vi "Auto Climb Loop.vi"() -> (1 "Winch Out":dbl, 2 "Fire":bool, 3 "Extend":bool)   [LabVIEW 2015]
uses:
  Common Code/Climb Presets.ctl
panel:
  in  "Climb Presets":T1
  in  "Climb?":bool=TRUE
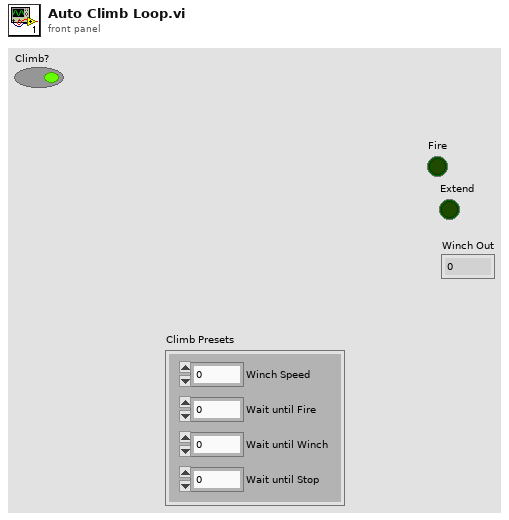
[diagram p1: front panel]
types:
  T1 = typedef "Climb Presets.ctl" = cluster{"Winch Speed":dbl, "Wait until Fire":dbl, "Wait until Winch":dbl, "Wait until Stop":dbl}
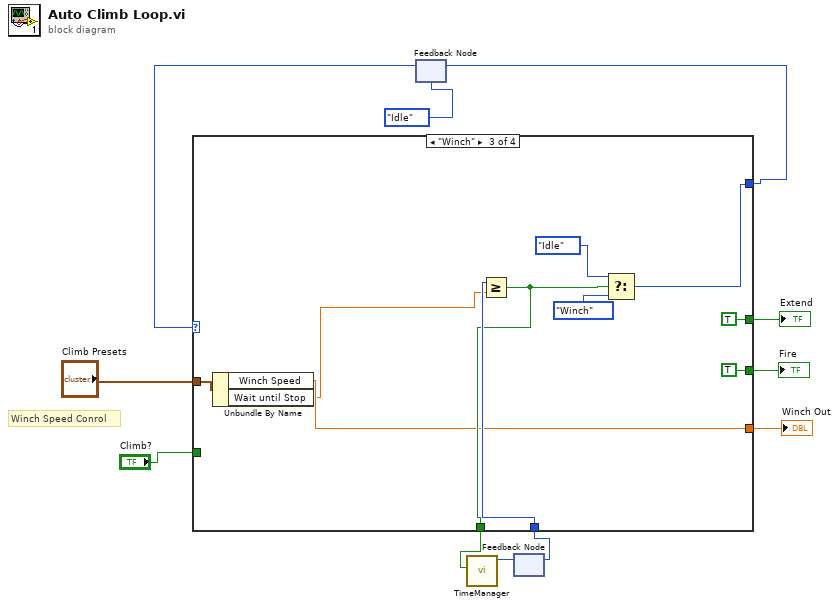
[diagram p0: block diagram]
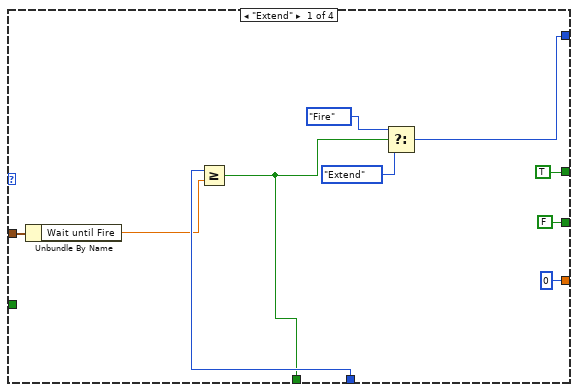
[diagram p2: hidden frame]
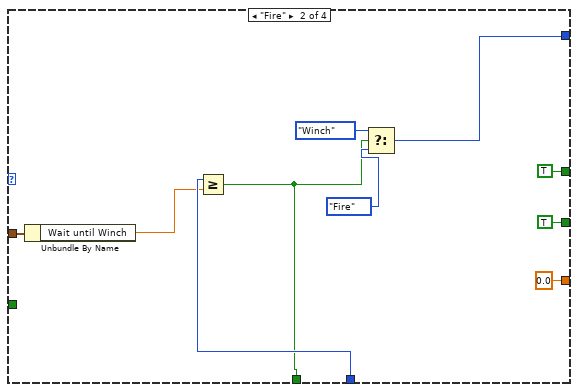
[diagram p3: hidden frame]
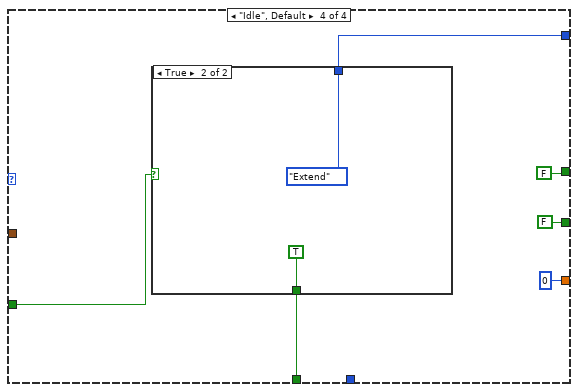
[diagram p4: hidden frame]
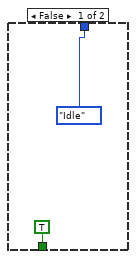
[diagram p5: hidden frame]
diagram:
  # "Winch Speed Conrol"
  n1 = feedback #1(enum16{"Extend", "Fire", "Winch", "Idle"}."Idle" ("Climb State")) -> (w11:enum16{"Extend", "Fire", "Winch", "Idle"})
  n2 = feedback #2() -> (w3:u32)  [unwired: 1 in]
  n3 = case shown="\"Winch\"" w11 {
    tunnel: [w17 w28 w39 w47] -> w9
    tunnel: [TRUE TRUE TRUE FALSE] -> w8
    tunnel: [FALSE TRUE TRUE FALSE] -> w7
    tunnel: [0 0.0 ("Winch Speed") w33 0] -> w6
    tunnel: [w14 w25 w35 w43] -> w5
    tunnel: w3 -> [w21 w31 w36 _]
    tunnel: "Climb?" -> [_ _ _ w42]
    tunnel: "Climb Presets" -> [w13 w23 w34 _]
    frame "Extend" {
      n4 = Unbundle By Name(w13) -> ("Wait until Fire"=w12:dbl)
      n5 = Greater Or Equal?(x=w21, y=w12) -> (x >= y?=w14:bool)
      n6 = Select(t=enum16{"Extend", "Fire", "Winch", "Idle"}."Fire" ("Climb State"), s=w14, f=enum16{"Extend", "Fire", "Winch", "Idle"}."Extend" ("Climb State")) -> (s? t:f=w17:enum16{"Extend", "Fire", "Winch", "Idle"})
    }
    frame "Fire" {
      n7 = Unbundle By Name(w23) -> ("Wait until Winch"=w22:dbl)
      n8 = Greater Or Equal?(x=w31, y=w22) -> (x >= y?=w25:bool)
      n9 = Select(t=enum16{"Extend", "Fire", "Winch", "Idle"}."Winch" ("Climb State"), s=w25, f=enum16{"Extend", "Fire", "Winch", "Idle"}."Fire" ("Climb State")) -> (s? t:f=w28:enum16{"Extend", "Fire", "Winch", "Idle"})
    }
    frame "Winch" {
      n10 = Unbundle By Name(w34) -> ("Winch Speed"=w33:dbl, "Wait until Stop"=w32:dbl)
      n11 = Greater Or Equal?(x=w36, y=w32) -> (x >= y?=w35:bool)
      n12 = Select(t=enum16{"Extend", "Fire", "Winch", "Idle"}."Idle" ("Climb State"), s=w35, f=enum16{"Extend", "Fire", "Winch", "Idle"}."Winch" ("Climb State")) -> (s? t:f=w39:enum16{"Extend", "Fire", "Winch", "Idle"})
    }
    frame "Idle", Default {
      n13 = case shown="True" w42 {
        tunnel: [enum16{"Extend", "Fire", "Winch", "Idle"}."Idle" ("Climb State") enum16{"Extend", "Fire", "Winch", "Idle"}."Extend" ("Climb State")] -> w47
        tunnel: [TRUE TRUE] -> w43
        frame False {
        }
        frame True {
        }
      }
    }
  }
  "Fire" <- w7
  "Winch Out" <- w6
  "Extend" <- w8
  n14 = feedback-in #1(w9) -> ()
  n15 = call "TimeManager.vi"("Reset?"=w5) -> ("Time Since Reset"=w4:u32)  [unwired: 9 in, 1 out]
  n16 = feedback-in #2(w4) -> ()
